vi "CPP-5168PuffReleaseAnalysis.vi"() -> (5 "Plug in titles":string[](array[string]), 7 "Plug in values":string[](array[string]))   [LabVIEW 2011]
uses:
  Controls/Post_Process.ctl
  Globals/Plug_in_data_global.vi
  Globals/Meas_global.vi
  <vilib>/measure/mascope.llb/Transition Measurements 1 chan.vi
  Globals/Dynamic_call_global.ph.vi
  <vilib>/measure/NI_MAPro.lvlib
panel:
  in  "PufferCard":tag="PXI1Slot3"
  out "FID2decayConstant":dbl
  out "FID1decayConstant":dbl
  in  "Valvetransition":u16(ring)=1 items=["falling", "rising"]
  out "FFID1 2":cluster{dbl, dbl, dbl[]}[](graph)
  out "Valve":cluster{dbl, dbl, dbl[]}(graph)
  in  "Averaging Samples":i32=1 min=1
  out "ValveShutAt":dbl format="%.2f"
  out "FFID2":T1(graph)
  out "Current Block No":i32
  out "FFID1":cluster{dbl, dbl, dbl[]}[](graph)
  out "SourceOffIndex":i32
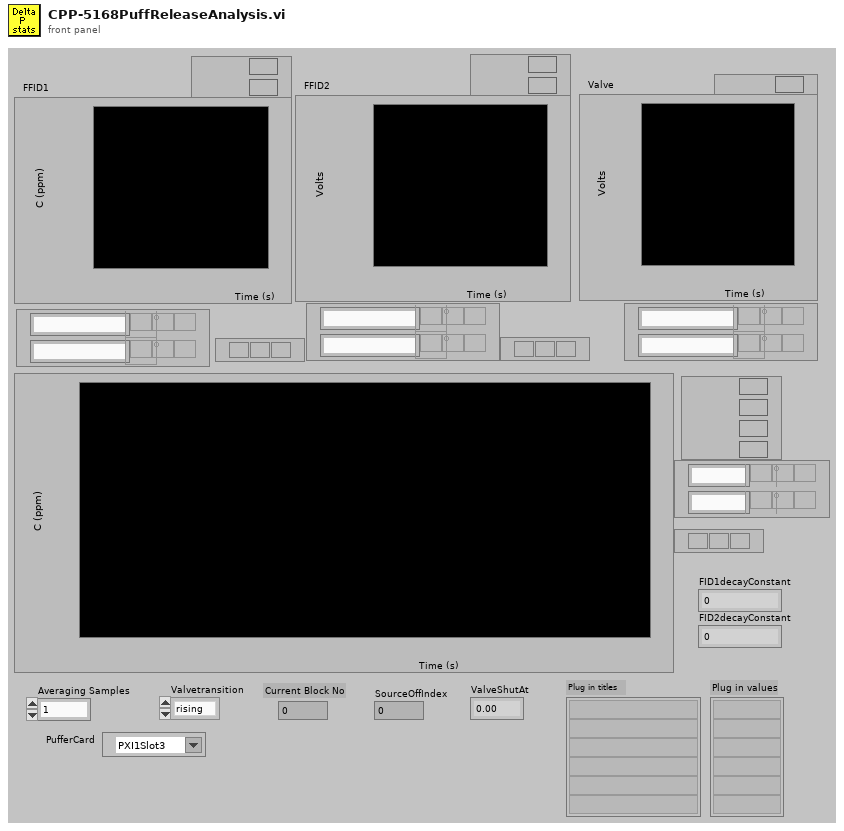
[diagram p1: front panel]
types:
  T1 = cluster{dbl, "SamplingRate":dbl, "Best Exponential Fit":dbl[]}[]
  T2 = enum16{"Save no data", "Save data in new files", "Save data in existing files"}
  T3 = typedef "Post_Process.ctl" = enum16{"Take New Data", "Post Process Raw Data File"}
  T4 = cluster{"start time":dbl, "end time":dbl, "ref levels":cluster{"high ref level":dbl, "mid ref level":dbl, "low ref level":dbl, "ref units":u16}}
  T5 = cluster{dbl, "SamplingRate":dbl, "Best Exponential Fit":dbl[]}
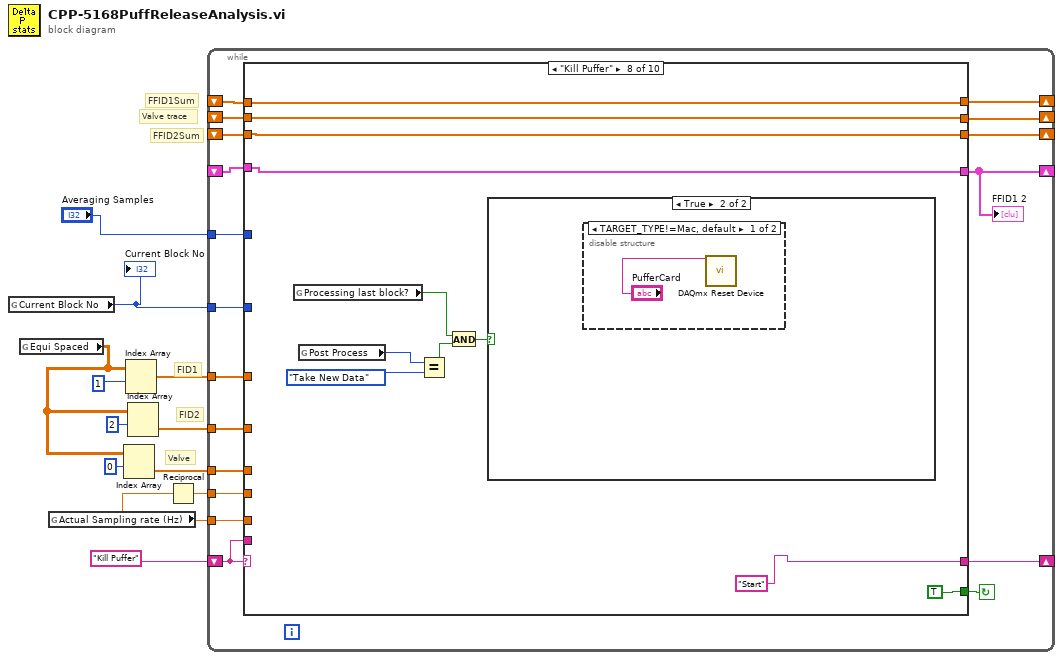
[diagram p0: block diagram]
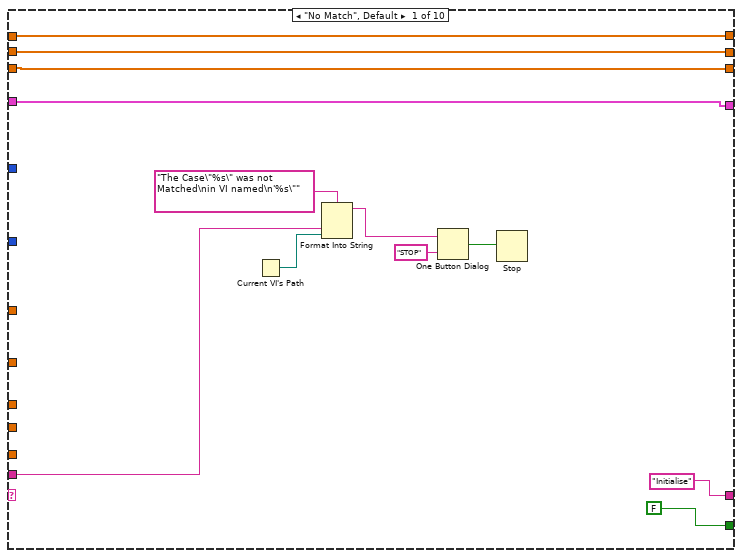
[diagram p2: hidden frame]
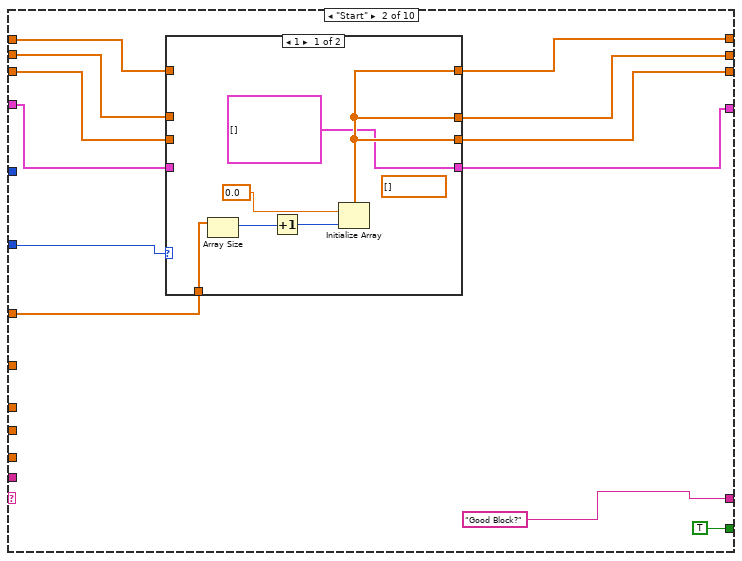
[diagram p3: hidden frame]
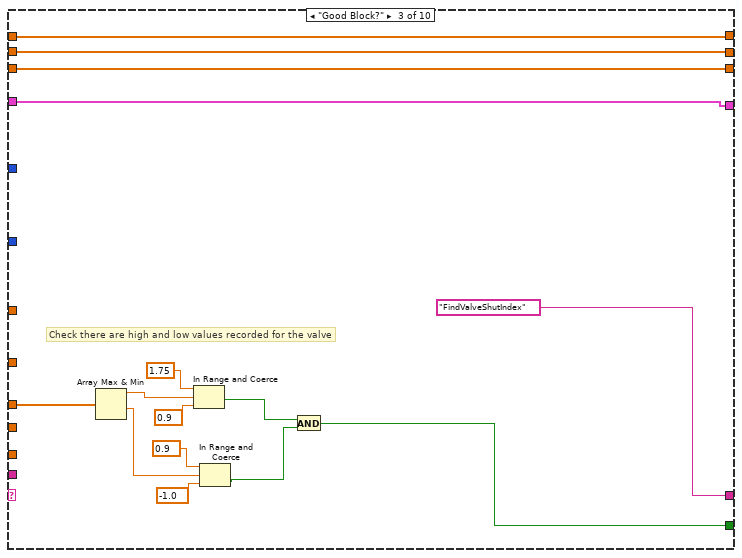
[diagram p5: hidden frame]
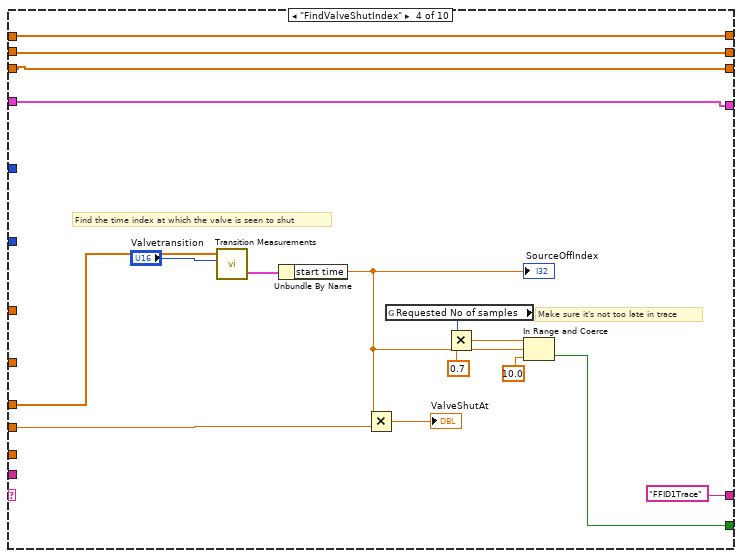
[diagram p6: hidden frame]
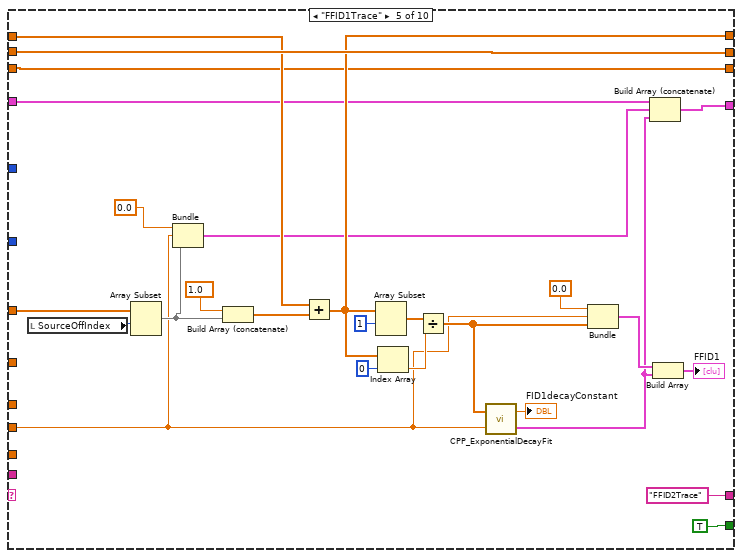
[diagram p7: hidden frame]
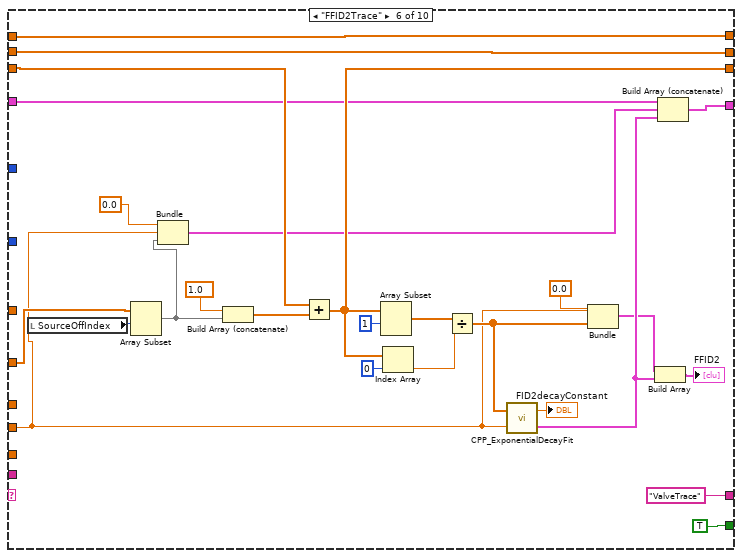
[diagram p8: hidden frame]
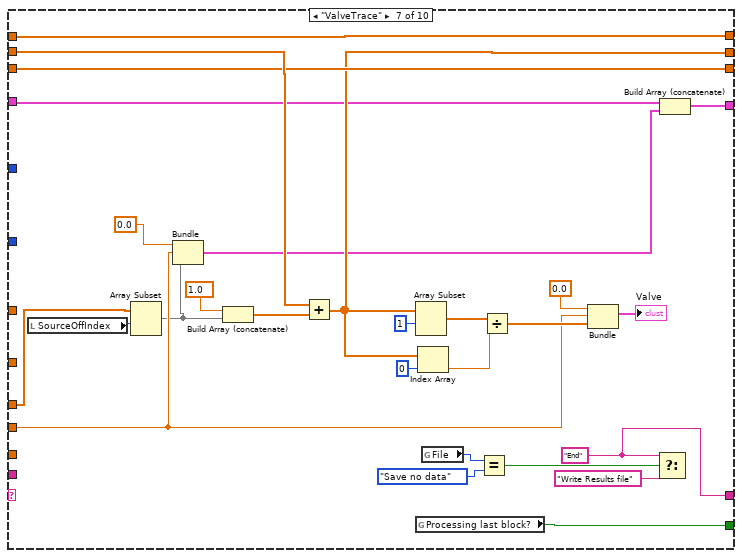
[diagram p9: hidden frame]
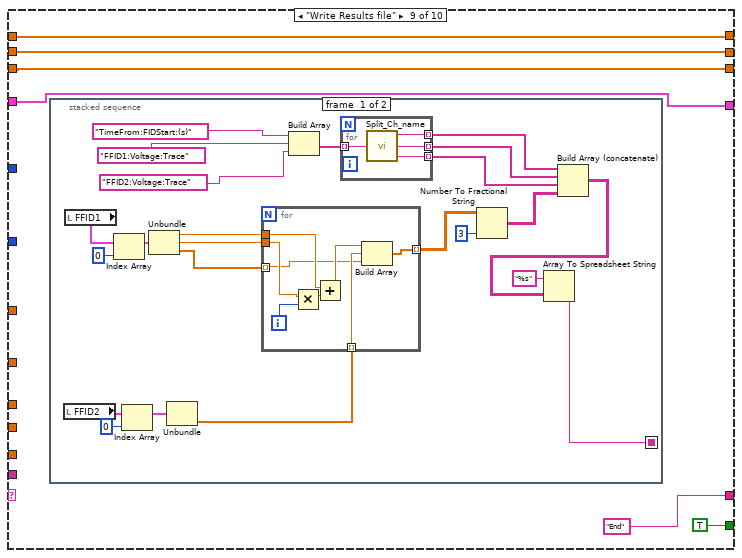
[diagram p12: hidden frame]
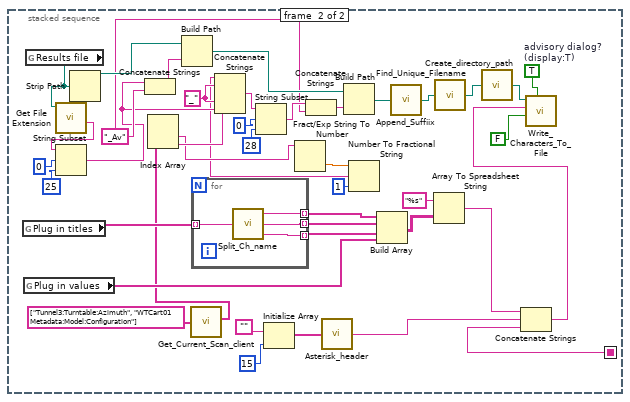
[diagram p13: hidden frame]
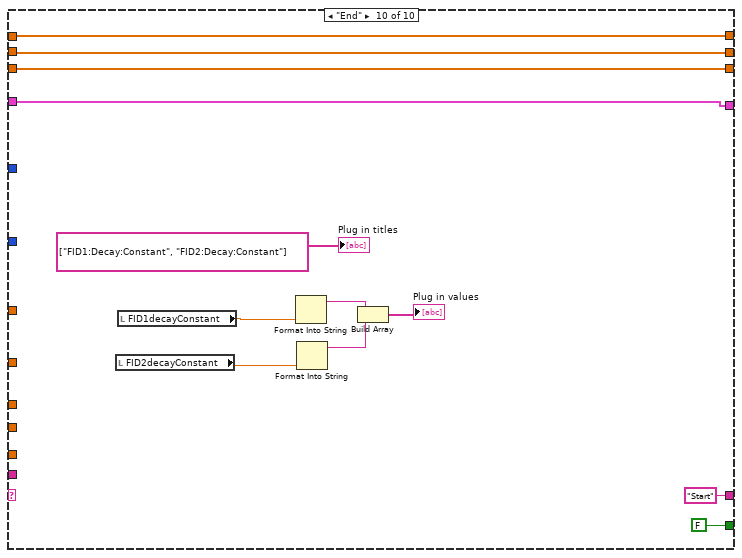
[diagram p14: hidden frame]
diagram:
  # "Valve"
  # "FID2"
  # "FID1"
  # "FFID2Sum"
  # "Valve trace"
  # "FFID1Sum"
  n1 = global read "Meas_global.vi" "Current Block No"() -> (w9:i32)
  "Current Block No" <- w9
  n2 = global read "Plug_in_data_global.vi" "Equi Spaced"() -> (w6:dbl[][])
  n3 = global read "Meas_global.vi" "Actual Sampling rate (Hz)"() -> (w2:dbl)
  n4 = Index Array(array=w6, index (row)=0) -> (element=w5:dbl[])  [unwired: 1 in]
  n5 = Index Array(array=w6, index (row)=1) -> (element=w10:dbl[])  [unwired: 1 in]
  n6 = Index Array(array=w6, index (row)=2) -> (element=w11:dbl[])  [unwired: 1 in]
  n7 = Reciprocal(x=w2) -> (1/x=w1:dbl)
  n8 = while {
    shift-left: "Kill Puffer" -> [w28]
    shift-right: [w29] -> _
    shift-right: [w27] -> _
    shift-left: _ -> [w24]
    shift-right: [w26] -> _
    shift-left: _ -> [w25]
    tunnel: w11 -> [w23]
    tunnel: w10 -> [w22]
    tunnel: w2 -> [w21]
    tunnel: w9 -> [w20]
    shift-right: [w18] -> _
    shift-left: _ -> [w17]
    tunnel: w5 -> [w19]
    tunnel: "Averaging Samples" -> [w16]
    tunnel: w1 -> [w15]
    shift-right: [w13] -> _
    shift-left: _ -> [w14]
    stop <- w30 continue-if-true
    n9 = case shown="\"Kill Puffer\"" w28 {
      tunnel: [FALSE TRUE ("Processing last block?") w74 w84 TRUE ("Processing last block?") TRUE ("Processing last block?") w153 TRUE ("Processing last block?") TRUE ("Processing last block?") FALSE ("Processing last block?")] -> w30
      tunnel: ["Initialise" "Good Block?" "FindValveShutIndex" "FFID1Trace" "FFID2Trace" "ValveTrace" w148 "Start" "End" "Start" ("f")] -> w29
      tunnel: w28 -> [w37 _ _ _ _ _ _ _ _ _]
      tunnel: [w34 w53 w79 w94 w111 w135 w165 w185 w192 w285] -> w27
      tunnel: [w33 w51 w78 w93 w119 w145 w162 w184 w191 w284] -> w26
      tunnel: w25 -> [w33 w50 w78 w93 w119 w145 w164 w184 w191 w284]
      tunnel: w24 -> [w34 w52 w79 w94 w117 w135 w165 w185 w192 w285]
      tunnel: w23 -> [_ _ _ _ _ w136 _ _ _ _]
      tunnel: w22 -> [_ w49 _ _ w118 _ _ _ _ _]
      tunnel: w21 -> [_ _ _ _ _ _ _ _ _ _]
      tunnel: w20 -> [_ w48 _ _ _ _ _ _ _ _]
      tunnel: w19 -> [_ _ w70 w89 _ _ w161 _ _ _]
      tunnel: [w32 w47 w71 w92 w108 w133 w163 w180 w188 w283] -> w18
      tunnel: w17 -> [w32 w46 w71 w92 w108 w134 w163 w180 w188 w283]
      tunnel: w16 -> [_ _ _ _ _ _ _ _ _ _]
      tunnel: w15 -> [_ _ _ w81 w98 w122 w156 _ _ _]
      tunnel: [w31 w44 w65 w80 w106 w132 w160 w176 w187 w280] -> w13
      tunnel: w14 -> [w31 w43 w65 w80 w107 w131 w159 w176 w187 w280]
      frame "No Match", Default {
        n10 = Current VI's Path() -> (path=w36:path)
        n11 = Format Into String(format string="The Case\"%s\" was not Matched\nin VI named\n'%s\"" ("Format String"), w37, w36) -> (resulting string=w40:string)  [unwired: 2 in, 1 out]
        n12 = One Button Dialog(message=w40, button name ("OK")="STOP") -> (true=w38:bool)
        n13 = Stop(stop? (T)=w38) -> ()
      }
      frame "Start" {
        n14 = case shown="1" w48 {
          tunnel: [w57 w64] -> w53
          tunnel: w52 -> [_ w64]
          tunnel: [w57 w63] -> w51
          tunnel: w50 -> [_ w63]
          tunnel: w49 -> [w60 _]
          tunnel: [w57 w62] -> w47
          tunnel: w46 -> [_ w62]
          tunnel: [cluster{dbl, dbl, dbl[]}[] [] w61] -> w44
          tunnel: w43 -> [_ w61]
          frame 1 {
            (unwired) dbl[] []
            n15 = Array Size(array=w60) -> (size(s)=w59:i32)
            n16 = Increment(x=w59) -> (x+1=w56:i32)
            n17 = Initialize Array(0.0 ("element"), w56) -> (w57:dbl[])
          }
          frame 2, Default {
          }
        }
      }
      frame "Good Block?" {
        # "Check there are high and low values recorded for the valve"
        n18 = Array Max & Min(array=w70) -> (max value=w73:dbl, min value=w67:dbl)  [unwired: 2 out]
        n19 = In Range and Coerce(upper limit=1.75, x=w73, lower limit=0.9 ("y")) -> (In Range?=w75:bool)  [unwired: 1 out]
        n20 = In Range and Coerce(upper limit=0.9, x=w67, lower limit=-1.0 ("y")) -> (In Range?=w66:bool)  [unwired: 1 out]
        n21 = And(x=w75, y=w66) -> (x .and. y?=w74:bool)
      }
      frame "FindValveShutIndex" {
        # "Make sure it's not too late in trace"
        # "Find the time index at which the valve is seen to shut"
        n22 = call-poly <vilib>:"Transition Measurements.vi"("polarity (rising)"="Valvetransition", "signal in"=w89) -> ("measurement info"=w90:T4)  [unwired: 4 in, 5 out]
        n23 = Unbundle By Name(w90) -> ("start time"=w83:dbl)
        "SourceOffIndex" <- w83
        n24 = Multiply(x=w83, y=w81) -> (x*y=→"ValveShutAt":dbl)
        n25 = global read "Meas_global.vi" "Requested No of samples"() -> (w88:i32)
        n26 = Multiply(x=w88, y=0.7 ("lower limit")) -> (x*y=w86:dbl)
        n27 = In Range and Coerce(upper limit=w86, x=w83, lower limit=10.0) -> (In Range?=w84:bool)  [unwired: 1 out]
      }
      frame "FFID1Trace" {
        n28 = local read "SourceOffIndex"() -> (w114:i32)
        n29 = Array Subset(array=w118, index=w114) -> (w104:dbl[])  [unwired: 1 in]
        n30 = Bundle(0.0, w98, w104) -> (w103:cluster{dbl, dbl, dbl[]})  [unwired: 1 out]
        n31 = Build Array (concatenate)(1.0, w104) -> (w115:dbl[])
        n32 = Add(x=w117, y=w115) -> (x+y=w111:dbl[])
        n33 = Array Subset(array=w111, index=1) -> (w110:dbl[])  [unwired: 1 in]
        n34 = Index Array(array=w111, index=0) -> (element=w109:dbl)
        n35 = Divide(x=w110, y=w109) -> (x/y=w102:dbl[])
        n36 = call "CPP_ExponentialDecayFit.vi"("SamplingRate"=w98, "DecayData"=w102) -> ("graphCluster"=w96:T5, "decayConstant"=→"FID1decayConstant":dbl)
        n37 = Bundle(0.0, w98, w102) -> (w101:cluster{dbl, dbl, dbl[]})  [unwired: 1 out]
        n38 = Build Array (concatenate)(w107, w103, w96) -> (w106:T1)
        n39 = Build Array(w101, w96) -> (→"FFID1":T1)
      }
      frame "FFID2Trace" {
        n40 = local read "SourceOffIndex"() -> (w142:i32)
        n41 = Array Subset(array=w136, index=w142) -> (w129:dbl[])  [unwired: 1 in]
        n42 = Bundle(0.0, w122, w129) -> (w128:cluster{dbl, dbl, dbl[]})  [unwired: 1 out]
        n43 = Build Array (concatenate)(1.0, w129) -> (w143:dbl[])
        n44 = Add(x=w134, y=w143) -> (x+y=w133:dbl[])
        n45 = Array Subset(array=w133, index=1) -> (w138:dbl[])  [unwired: 1 in]
        n46 = Index Array(array=w133, index=0) -> (element=w137:dbl)
        n47 = Divide(x=w138, y=w137) -> (x/y=w123:dbl[])
        n48 = call "CPP_ExponentialDecayFit.vi"("SamplingRate"=w122, "DecayData"=w123) -> ("graphCluster"=w126:T5, "decayConstant"=→"FID2decayConstant":dbl)
        n49 = Bundle(0.0, w122, w123) -> (w125:cluster{dbl, dbl, dbl[]})  [unwired: 1 out]
        n50 = Build Array(w125, w126) -> (→"FFID2":T1)
        n51 = Build Array (concatenate)(w131, w128, w126) -> (w132:T1)
      }
      frame "ValveTrace" {
        w148 = "End"
        n52 = local read "SourceOffIndex"() -> (w172:i32)
        n53 = Array Subset(array=w161, index=w172) -> (w155:dbl[])  [unwired: 1 in]
        n54 = Bundle(0.0, w156, w155) -> (w154:cluster{dbl, dbl, dbl[]})  [unwired: 1 out]
        n55 = Build Array (concatenate)(1.0, w155) -> (w173:dbl[])
        n56 = Add(x=w164, y=w173) -> (x+y=w162:dbl[])
        n57 = Array Subset(array=w162, index=1) -> (w167:dbl[])  [unwired: 1 in]
        n58 = global read "Meas_global.vi" "Processing last block?"() -> (w153:bool)
        n59 = Index Array(array=w162, index=0) -> (element=w166:dbl)
        n60 = global read "Meas_global.vi" "File"() -> (w152:T2)
        n61 = Equal?(x=w152, y=T2."Save no data" ("File")) -> (x = y?=w149:bool)
        n62 = Divide(x=w167, y=w166) -> (x/y=w171:dbl[])
        n63 = Bundle(0.0, w156, w171) -> (→"Valve":cluster{dbl, dbl, dbl[]})  [unwired: 1 out]
        n64 = Select(t=w148, s=w149, f="Write Results file") -> ()  [unwired: 1 out]
        n65 = Build Array (concatenate)(w159, w154) -> (w160:T1)
      }
      frame "Kill Puffer" {
        n66 = global read "Meas_global.vi" "Processing last block?"() -> (w179:bool)
        n67 = global read "Meas_global.vi" "Post Process"() -> (w182:T3)
        n68 = Equal?(x=w182, y=Post_Process."Take New Data" ("Post Process")) -> (x = y?=w178:bool)
        n69 = And(x=w179, y=w178) -> (x .and. y?=w177:bool)
        n70 = case shown="True" w177 {
          frame False {
          }
          frame True {
            n71 = disable-structure shown="TARGET_TYPE!=Mac, default" {
              frame condition #0 (active) {
                n72 = call <vilib>:"DAQmx Reset Device.vi"("device in"="PufferCard") -> ()  [unwired: 14 in, 1 out]
              }
              frame condition #1 {
              }
            }
          }
        }
      }
      frame "Write Results file" {
        n73 = stacked-sequence {
          seq-local: [w205 _] -> [_ w255]
          frame #0 {
            n74 = local read "FFID2"() -> (w204:T1)
            n75 = local read "FFID1"() -> (w215:cluster{dbl, dbl, dbl[]}[])
            n76 = Index Array(array=w215, index=0) -> (element=w196:cluster{dbl, dbl, dbl[]})
            n77 = Index Array(array=w204, index=0) -> (element=w194:T5)
            n78 = Unbundle(w196) -> (w213:dbl, w214:dbl, w212:dbl[])
            n79 = Unbundle(w194) -> ("Best Exponential Fit"=w203:dbl[])  [unwired: 2 out]
            n80 = for {
              tunnel: w214 -> [w226]
              tunnel: w213 -> [w225]
              tunnel: w212 -> [w220] mode=indexing
              tunnel: [w223] -> w210 mode=indexing
              tunnel: w203 -> [w221] mode=indexing
              i -> [w227]
              n81 = Multiply(x=w226, y=w227) -> (x*y=w224:dbl)
              n82 = Add(x=w225, y=w224) -> (x+y=w222:dbl)
              n83 = Build Array(w222, w221, w220) -> (w223:dbl[])
            }
            n84 = Build Array("TimeFrom:FIDStart:(s)", "FFID1:Voltage:Trace", "FFID2:Voltage:Trace") -> (w200:string[])
            n85 = for {
              tunnel: w200 -> [w219] mode=indexing
              tunnel: [w218] -> w199 mode=indexing
              tunnel: [w217] -> w198 mode=indexing
              tunnel: [w216] -> w197 mode=indexing
              n86 = call "Split_Ch_name.vi"("Ch name"=w219) -> ("Top level"=w218:string, "Middle"=w217:string, "Low level"=w216:string)
            }
            n87 = Number To Fractional String(number=w210, precision (6)=i16 3) -> (F-format string=w209:string[][])  [unwired: 2 out]
            n88 = Build Array (concatenate)(w199, w198, w197, w209) -> (w207:string[][])
            n89 = Array To Spreadsheet String(array=w207, 3:"%s" ("format string")) -> (spreadsheet string=w205:string)  [unwired: 1 out]
          }
          frame #1 {
            w243 = "_" ("string")
            w269 = TRUE  # advisory dialog? (display:T)
            w239 = "_Av" ("string")
            n90 = global read "Dynamic_call_global.ph.vi" "Plug in titles"() -> (w267:string[])
            n91 = global read "Dynamic_call_global.ph.vi" "Plug in values"() -> (w263:string[])
            n92 = global read "Meas_global.vi" "Results file"() -> (w249:path)
            n93 = call <vilib>:"Get File Extension.vi"("file"=w249) -> ("filename without extension"=w235:string)  [unwired: 7 in, 3 out]
            n94 = String Subset(string=w235, offset (0)=0, length (rest)=25 ("length (rest)")) -> (substring=w234:string)
            n95 = Strip Path(path=w249) -> (stripped path=w248:path)  [unwired: 1 out]
            n96 = Concatenate Strings(w234, w239) -> (w246:string)
            n97 = Build Path(base path=w248, name or relative path=w246) -> (appended path=w247:path)
            n98 = call "Get_Current_Scan_client.vi"("ADAM Ch Names"=string[] ["Tunnel3:Turntable:Azimuth", "WTCart01 Metadata:Model:Configuration"]) -> ("String values"=w244:string[])  [unwired: 1 in, 2 out]
            n99 = Index Array(array=w244) -> (element #1=w231:string, element #2=w242:string)  [unwired: 2 in]
            n100 = for {
              tunnel: w267 -> [w273] mode=indexing
              tunnel: [w272] -> w266 mode=indexing
              tunnel: [w271] -> w265 mode=indexing
              tunnel: [w270] -> w264 mode=indexing
              n101 = call "Split_Ch_name.vi"("Ch name"=w273) -> ("Top level"=w272:string, "Middle"=w271:string, "Low level"=w270:string)
            }
            n102 = Initialize Array("", 15) -> (w260:string[])
            n103 = Fract/Exp String To Number(string=w231) -> (number=w230:dbl)  [unwired: 3 in, 1 out]
            n104 = call "Asterisk_header.vi"("Channel names"=w260) -> ("Header string"=w256:string)
            n105 = Number To Fractional String(number=w230, precision (6)=i16 1) -> (F-format string=w228:string)  [unwired: 2 in]
            n106 = Concatenate Strings(w228, w243, w242, w243, w234) -> (w241:string)
            n107 = String Subset(string=w241, offset (0)=0, length (rest)=28 ("length (rest)")) -> (substring=w240:string)
            n108 = Concatenate Strings(w240, w239) -> (w238:string)
            n109 = Build Path(base path=w247, name or relative path=w238) -> (appended path=w251:path)
            n110 = Build Array(w266, w265, w264, w263) -> (w261:string[][])
            n111 = call "Append_Suffiix.vi"("Results file"=w251) -> ("appended path"=w250:path)
            n112 = Array To Spreadsheet String(array=w261, 3:"%s" ("format string")) -> (spreadsheet string=w257:string)  [unwired: 1 out]
            n113 = call "Find_Unique_Filename.vi"("Path In"=w250) -> ("Unique Path Out"=w233:path)  [unwired: 1 in, 1 out]
            n114 = call "Create_directory_path.vi"("Path name"=w233) -> ("Path name Out"=w232:path)
            n115 = Concatenate Strings(w257, w256, w255) -> (w254:string)
            n116 = call "Write_Characters_To_File.vi"("file path (dialog if empty)"=w232, "advisory dialog? (display:T)"=w269, "character string"=w254, "append to file? (new file:F)"=FALSE) -> ()  [unwired: 1 in, 4 out]
          }
        }
      }
      frame "End" {
        n117 = local read "FID2decayConstant"() -> (w276:dbl)
        n118 = local read "FID1decayConstant"() -> (w278:dbl)
        n119 = Format Into String(w278) -> (resulting string=w277:string)  [unwired: 3 in, 1 out]
        n120 = Format Into String(w276) -> (resulting string=w275:string)  [unwired: 3 in, 1 out]
        n121 = Build Array(w277, w275) -> (→"Plug in values":string[])
        "Plug in titles" <- string[] ["FID1:Decay:Constant", "FID2:Decay:Constant"] ("Plug in titles")
      }
    }
    "FFID1 2" <- w13
  }
